vi "Stationary Characters.vi"(11 "Main Picture in":picture) -> (3 "Main Picture out":picture)   [LabVIEW 2014]
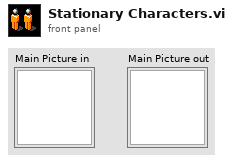
[diagram p1: front panel]
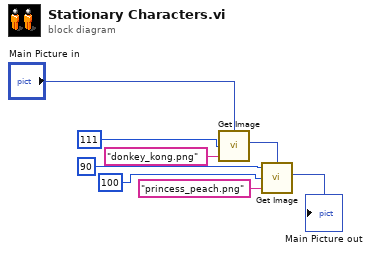
[diagram p0: block diagram]
diagram:
  n1 = call "Get Image.vi"("Input Picture"="Main Picture in", "String"="donkey_kong.png", "Bottom"=111) -> ("Main Picture"=w4:picture)  [unwired: 1 in]
  n2 = call "Get Image.vi"("Input Picture"=w4, "String"="princess_peach.png", "Bottom"=100, "Left"=90) -> ("Main Picture"=→"Main Picture out":picture)
